vi "Get Project Package Version.vi"(10 "Template Project":path, 11 "Project Path":path) -> (0 "Template Vers Str":string, 1 "Project Vers Str":string, 2 "Template Version":T1, 3 "Project Version":T1)   [LabVIEW 2020]
uses:
  Version.ctl
  Tags.ctl
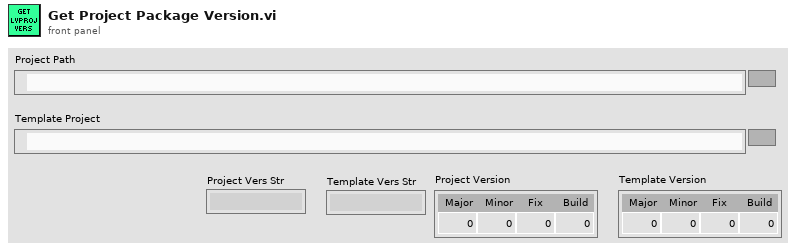
[diagram p1: front panel]
types:
  T1 = typedef "Version.ctl" = cluster{"Major":u16, "Minor":u16, "Fix":u16, "Build":u16}
  T2 = typedef "Tags.ctl" = enum16{"sol.reversi.version"}
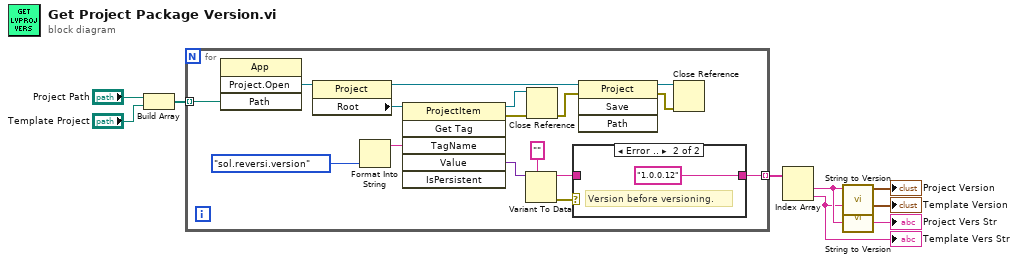
[diagram p0: block diagram]
diagram:
  n1 = Build Array("Project Path", "Template Project") -> (w6:path[])
  n2 = for {
    tunnel: [w11] -> w8 mode=indexing
    tunnel: w6 -> [w14] mode=indexing
    n3 = invoke class="App" method="Project.Open"("Path"=w14) -> ("Project:Open"=w24:refnum<vi>)  [unwired: 3 in, 3 out]
    n4 = property class="Project"(reference=w24) -> (reference out=w23:refnum<vi>, "Root"=w22:refnum<vi>)  [unwired: 1 in, 1 out]
    n5 = Format Into String(Tags."sol.reversi.version" ("Tags")) -> (resulting string=w9:string)  [unwired: 3 in, 1 out]
    n6 = invoke class="ProjectItem" method="Get Tag"(reference=w22, "TagName"=w9) -> (reference out=w20:refnum<vi>, error out=w19:errorcluster, "Value"=w16:variant)  [unwired: 4 in, 3 out]
    n7 = Variant To Data(type="", Variant=w16) -> (data=w12:string, error out=w13:errorcluster)  [unwired: 1 in]
    n8 = Close Reference(reference=w20, error in (no error)=w19) -> (error out=w18:errorcluster)
    n9 = case shown="Error .." w13 {
      tunnel: w12 -> [w25 _]
      tunnel: [w25 "1.0.0.12"] -> w11
      frame No Error {
      }
      frame Error {
        # "Version before versioning."
      }
    }
    n10 = invoke class="Project" method="Save"(reference=w23, error in=w18) -> (reference out=w21:refnum<vi>, error out=w17:errorcluster)  [unwired: 2 in, 2 out]
    n11 = Close Reference(reference=w21, error in (no error)=w17) -> ()  [unwired: 1 out]
  }
  n12 = Index Array(array=w8) -> (element #1=w4:string, element #2=w1:string)  [unwired: 2 in]
  "Project Vers Str" <- w4
  "Template Vers Str" <- w1
  n13 = call "String to Version.vi"("String Version"=w4) -> ("Version"=→"Project Version":T1)  [unwired: 10 in]
  n14 = call "String to Version.vi"("String Version"=w1) -> ("Version"=→"Template Version":T1)  [unwired: 10 in]
